vi "GVZwischenspeicher.vi"() -> ()   [LabVIEW 2017]
panel:
  in  "read":string[](array[string])
  in  "write":string[](array[string])
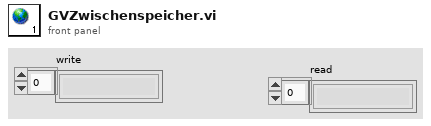
[diagram p1: front panel]
diagram:
